vi "Read from Hardware.vi"(8 "error in (no error)":errorcluster, 10 "Values in":dbl[](array[numeric]), 11 "NI-XNET CAN Reader Execution Unit in":refnum<class "NI-XNET CAN Reader Execution Unit.lvclass">) -> (0 "error out":errorcluster, 2 "Values out":dbl[](array[numeric]), 3 "NI-XNET CAN Reader Execution Unit out":refnum<class "NI-XNET CAN Reader Execution Unit.lvclass">)   [LabVIEW 2020, in "Communication Bus Template Engine.lvlib" / "Implementation.lvlib" / "NI-XNET CAN Reader Execution Unit.lvclass"]
uses:
  NI-XNET CAN Reader Execution Unit.lvclass
  <vilib>/xnet/xnet.llb/XNET Read (Signal Single-point).vi
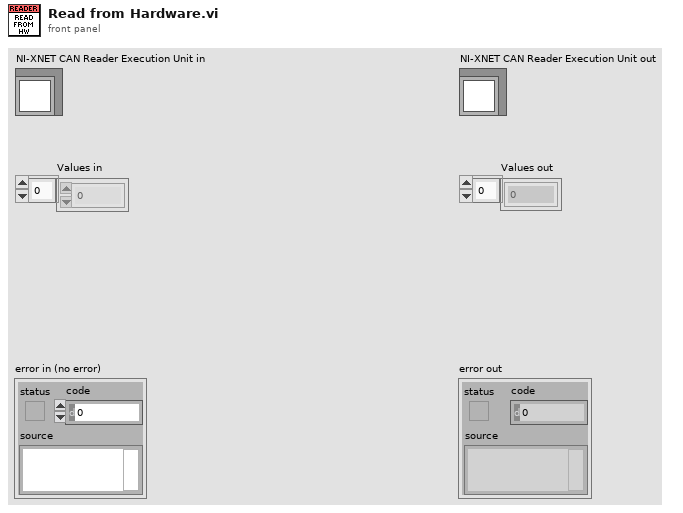
[diagram p1: front panel]
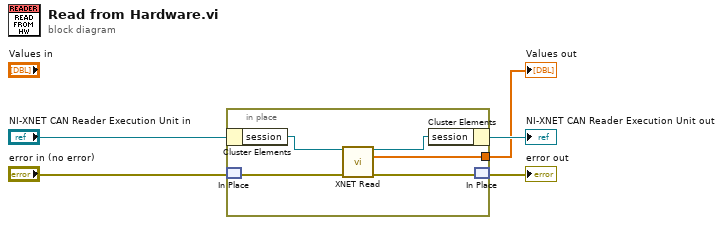
[diagram p0: block diagram]
diagram:
  n1 = in-place {
    in-place-border: [w6] -> w1
    n2 = in-place-cluster #1("NI-XNET CAN Reader Execution Unit in") -> ("session"=w10:refnum<k21>)
    n3 = in-place-match #2("error in (no error)") -> (w8:errorcluster)
    n4 = call-poly <vilib>:"XNET Read.vi"("session in"=w10, "error in (no error)"=w8) -> ("session out"=w7:refnum<k21>, "data"=w6:dbl[], "error out"=w9:errorcluster)  [unwired: 11 in]
    n5 = in-place-cluster #1("session"=w7) -> (→"NI-XNET CAN Reader Execution Unit out":refnum<class "NI-XNET CAN Reader Execution Unit.lvclass">)
    n6 = in-place-match #2(w9) -> (→"error out":errorcluster)
  }
  "Values out" <- w1
